vi "SetProperty.vi"(6 "Data":u32, 7 "Set":bool, 8 "error in (no error)":errorcluster, 9 "SubIndex":u8, 10 "Index":u16, 11 "Template SoftMotion Drive Interface Plug-in Class in":refnum<class "Template SoftMotion Drive Interface Plug-in Class.lvclass">) -> (0 "error out":errorcluster, 2 "Done":bool, 3 "Template SoftMotion Drive Interface Plug-in Class out":refnum<class "Template SoftMotion Drive Interface Plug-in Class.lvclass">)   [LabVIEW 2014, in "Template SoftMotion Drive Interface Plug-in Class.lvclass"]
uses:
  Template SoftMotion Drive Interface Plug-in Class.lvclass
  <vilib>/Motion/plugins/PluginFramework/nismPluginAxisBase/nismPluginAxisBaseClass.lvclass
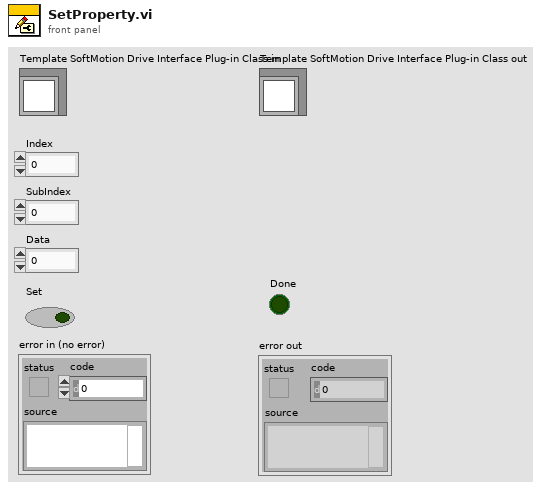
[diagram p1: front panel]
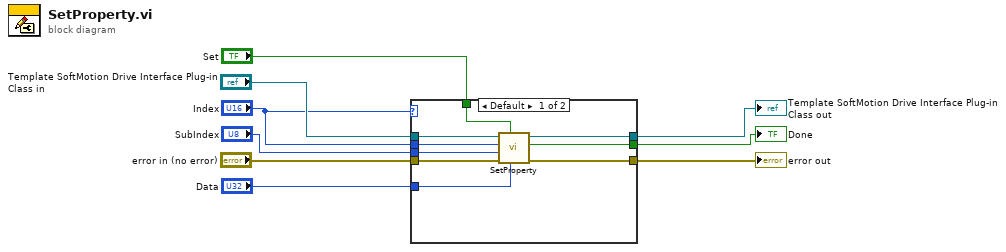
[diagram p0: block diagram]
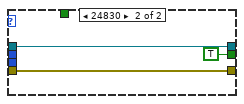
[diagram p2: hidden frame]
diagram:
  n1 = case shown="Default" "Index" {
    tunnel: [w18 w19] -> w9
    tunnel: [w17 TRUE ("Done")] -> w8
    tunnel: [w16 w21] -> w7
    tunnel: "Data" -> [w15 _]
    tunnel: "Set" -> [w14 _]
    tunnel: "error in (no error)" -> [w13 w19]
    tunnel: "SubIndex" -> [w12 _]
    tunnel: "Index" -> [w11 _]
    tunnel: "Template SoftMotion Drive Interface Plug-in Class in" -> [w10 w21]
    frame Default {
      n2 = call-parent "SetProperty.vi"("Data"=w15, "Set"=w14, "error in (no error)"=w13, "SubIndex"=w12, "Index"=w11, "nismPluginAxisBaseClass in"=w10) -> ("error out"=w18:errorcluster, "Done"=w17:bool, "nismPluginAxisBaseClass out"=w16:refnum<class "Template SoftMotion Drive Interface Plug-in Class.lvclass">)  [unwired: 3 in]
    }
    frame 24830 {
    }
  }
  "error out" <- w9
  "Template SoftMotion Drive Interface Plug-in Class out" <- w7
  "Done" <- w8
